vi "Cleanup.vi"(8 "error in (no error)":errorcluster, 11 "CDependencyList in":refnum<class "CDependencyList.lvclass">) -> (0 "error out":errorcluster, 3 "CDependencyList out":refnum<class "CDependencyList.lvclass">)   [LabVIEW 2020, in "DependencyInspection.lvlib" / "CDependencyList.lvclass"]
uses:
  CDependencyList.lvclass
  obj/Addons/LabVIEWObjectInterfaces.lvlibp/LabVIEWObjectInterfaces/ILabVIEWItem/ILabVIEWItem.lvclass
  DependencyList.ctl
  QualifiedNamesToPathsMap.ctl
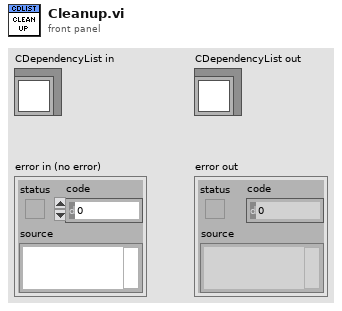
[diagram p1: front panel]
types:
  T1 = typedef "DependencyInspection.lvlib/CDependencyList.lvclass/QualifiedNamesToPathsMap.ctl" = map{string, string}
  T2 = typedef "DependencyInspection.lvlib/CDependencyList.lvclass/DependencyList.ctl" = map{string, refnum<class "ILabVIEWItem.lvclass">}
  T3 = typedef "DependencyInspection.lvlib/CDependencyList.lvclass/DependencyListRef.ctl" = refnum<data-value>
  T4 = typedef "DependencyInspection.lvlib/CDependencyList.lvclass/QualifiedNamesToPathsMapRef.ctl" = refnum<data-value>
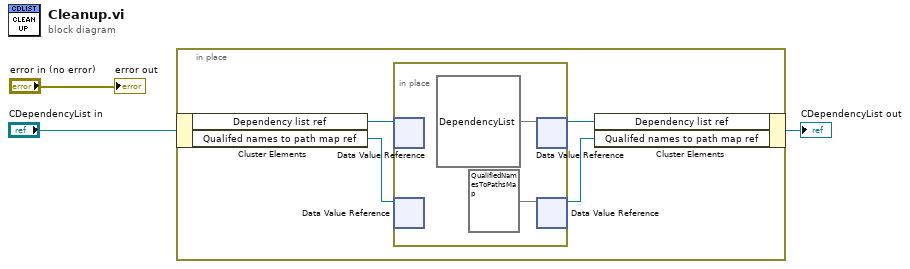
[diagram p0: block diagram]
diagram:
  n1 = in-place {
    n2 = in-place-cluster #1("CDependencyList in") -> ("Dependency list ref"=w7:T3, "Qualifed names to path map ref"=w6:T4)
    n3 = in-place {
      n4 = in-place-dvr #2(w7) -> ()  [unwired: 2 out]
      n5 = in-place-dvr #3(w6) -> ()  [unwired: 2 out]
      n6 = in-place-dvr #2(T2 {} ("data value")) -> (w5:T3)  [unwired: 1 out]
      n7 = in-place-dvr #3(T1 {} ("data value")) -> (w4:T4)  [unwired: 1 out]
    }
    n8 = in-place-cluster #1("Dependency list ref"=w5, "Qualifed names to path map ref"=w4) -> (→"CDependencyList out":refnum<class "CDependencyList.lvclass">)
  }
  "error out" <- "error in (no error)"
